vi "actuationIT6412w2110.vi"() -> ()   [LabVIEW 2023]
uses:
  IT64001/IT6400.lvlib
panel:
  out "error out 5":errorcluster
  in  "stop 5":bool
  out "Voltage 6":cluster{"Y":dbl[], "Y":dbl[]}[](graph)
  out "Voltage 6":dbl[](graph)
  out "Voltage 6":dbl[](array[numeric])
  out "error out 4":errorcluster
  out "Current time 4":timestamp
  in  "error in (no error) 3":errorcluster
  in  "VISA 2110 for voltage":refnum<visa-resource-name>
  out "Current through 330 ohm resistor'/mA 3":cluster{"Y":dbl[], "Y":dbl[]}[](graph)
  out "Voltage across 330 ohm resistor' 5":dbl[](graph)
  out "Voltage across 330 ohm resistor' 4":dbl[](array[numeric])
  in  "Filename 4":path caption="Filename"
  in  "Volt (0 V) 3":dbl min=-15.0 max=15.0 format="%.3g"
  in  "On/Off 3":bool
  in  "Pause/ms 3":i32=20
  out "Actual Voltage Level (V) 3":dbl[](array[numeric])
  out "Voltage'/V 3":dbl[](graph)
  in  "stop 3":bool
  out "Voltage'/V 2":cluster{"Y":dbl[], "Y":dbl[]}[](graph)
  in  "Filename 3":path caption="Filename"
  out "Current time 3":timestamp
  in  "period/s 2":i32
  in  "Boolean 2":bool
  in  "on time 2":dbl format="%#_13g"
  out "Voltage across 330 ohm resistor' 3":dbl[](array[numeric])
  out "Voltage across 330 ohm resistor' 2":dbl[](graph)
  out "Current through 330 ohm resistor'/mA 2":cluster{"Y":dbl[], "Y":dbl[]}[](graph)
  out "Current through 330 ohm resistor'/mA":cluster{"Y":dbl[], "Y":dbl[]}[](graph)
  out "Voltage across 330 ohm resistor'":dbl[](graph)
  out "Voltage across 330 ohm resistor'":dbl[](array[numeric])
  in  "Volt (0 V) 2":dbl min=-15.0 max=15.0 format="%.3g"
  in  "On/Off 2":bool
  in  "Pause/ms 2":i32=20
  out "Actual Voltage Level (V) 2":dbl[](array[numeric])
  out "Voltage'/V":dbl[](graph)
  in  "stop 2":bool
  out "Voltage'/V":cluster{"Y":dbl[], "Y":dbl[]}[](graph)
  in  "Filename 2":path caption="Filename"
  out "Current time 2":timestamp
  in  "period/s":i32
  in  "Boolean":bool
  in  "on time":dbl format="%#_13g"
  in  "Freq Sweep (1)\nCyclic voltammetry (2)\nSigGen (3)":i32 min=0 max=3 step=1
  in  "Camera":bool=TRUE
  out "Start time":timestamp
  out "current through 330ohm resistor/mA":cluster{"Y":dbl[], "Y":dbl[]}[](graph)
  out "Voltage across 330 ohm resistor":dbl[](graph)
  out "voltage across 330ohm resistor/V":dbl[](array[numeric])
  out "error out 3":errorcluster
  in  "error in (no error) 2":errorcluster
  in  "VISA 2110 for current":refnum<visa-resource-name>
  out "Timer":dbl
  in  "Countdown/s":i32=3
  out "Current time":timestamp
  in  "Filename":path
  out "Voltage/V":cluster{"Y":dbl[], "Y":dbl[]}[](graph)
  in  "stop":bool
  in  "Pause/ms":i32=100
  out "Voltage/V":dbl[](graph)
  out "Actual Voltage Level (V)":dbl[](array[numeric])
  in  "Sign":bool=TRUE
  in  "On/Off":bool
  in  "Volt (0 V)":dbl min=-15.0 max=15.0 format="%.3g"
  in  "Volt Limit (0 V)":dbl=9.0 min=0.0 max=15.0 format="%.3g"
  in  "Enable Volt Lim (T: Enable)":bool=TRUE
  in  "Curr Limit (0 A)":dbl=1.0 min=0.0 format="%.3g"
  in  "Enable Curr Lim (T: Enable)":bool=TRUE
  in  "Channel":i32=1 min=1 max=2
  in  "VOLT Range (0.0 v)":dbl=9.0 min=0.0 max=15.0 format="%.2g"
  in  "Enable OVP (T: Enable)":bool=TRUE
  in  "Reset":bool
  in  "Serial Configuration":T1={"Baud Rate"=9600, "Parity"=0, "Data Bits"=8, "Stop Bits"=10} {"Stop Bits" items=["1.0"=10, "1.5"=15, "2.0"=20]; "Data Bits" items=["7"=7, "8"=8]; "Parity" items=["None", "Odd", "Even", "Mark", "Space"]; "Baud Rate" items=["300"=300, "600"=600, "1200"=1200, "2400"=2400, "4800"=4800, "9600"=9600, "19200"=19200]}
  in  "Local/\nRemote":bool caption="Local/Remote"
  out "VISA resource name out":refnum<visa-resource-name>
  out "error out":errorcluster
  in  "error in (no error)":errorcluster
  in  "VISA resource name":refnum<visa-resource-name>
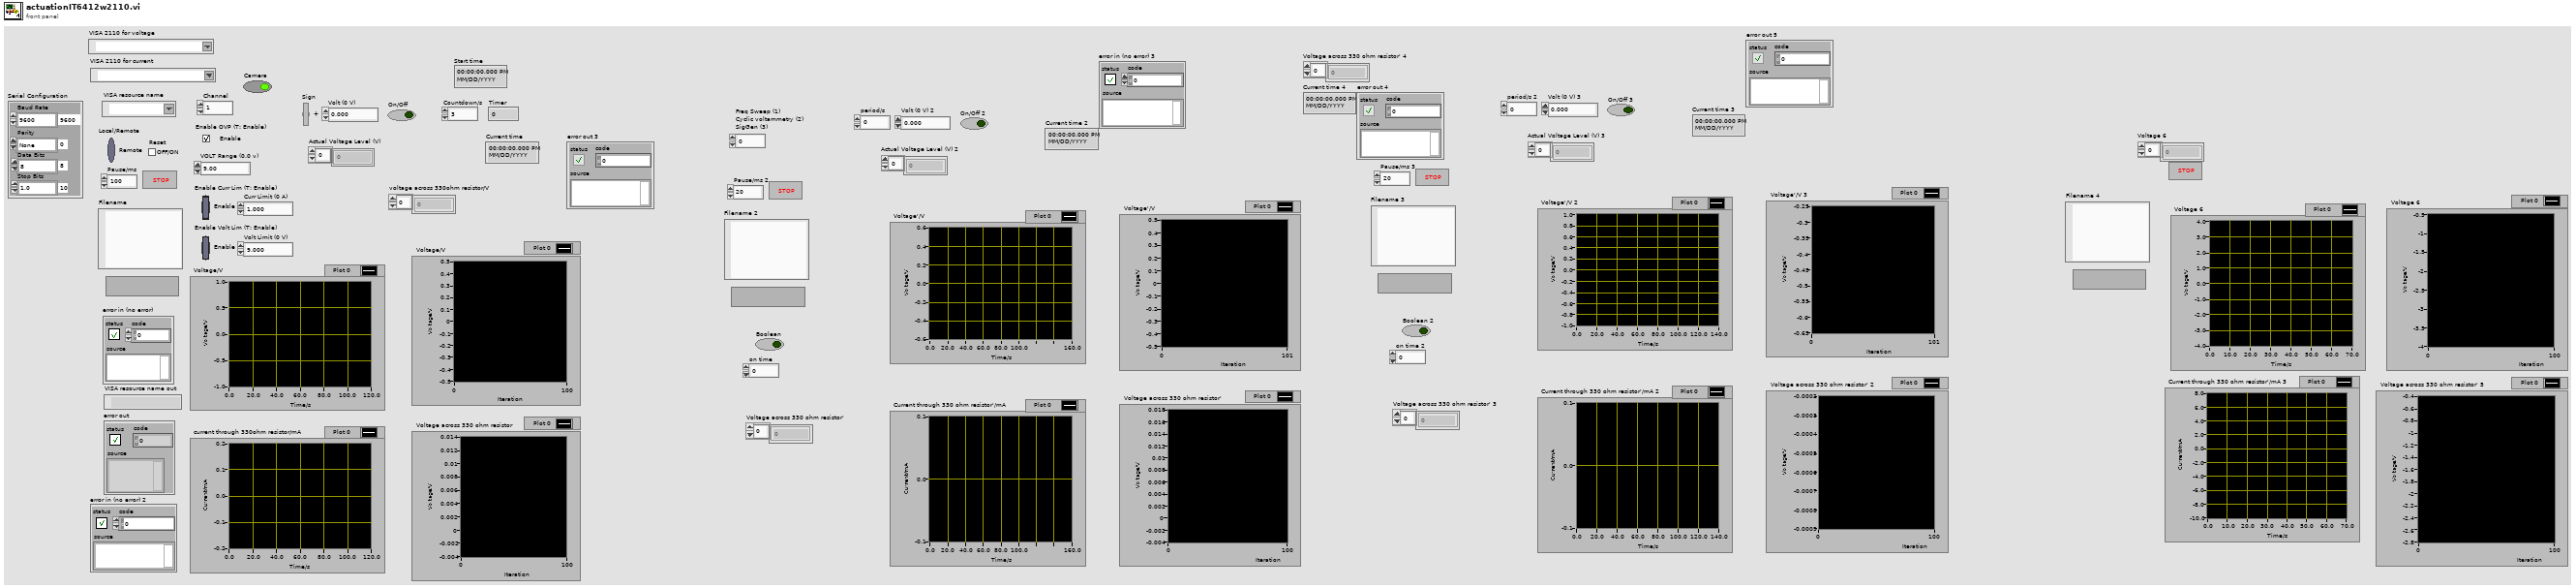
[diagram p1: front panel]
types:
  T1 = cluster{"Baud Rate":u32, "Parity":u16, "Data Bits":u16, "Stop Bits":u16}
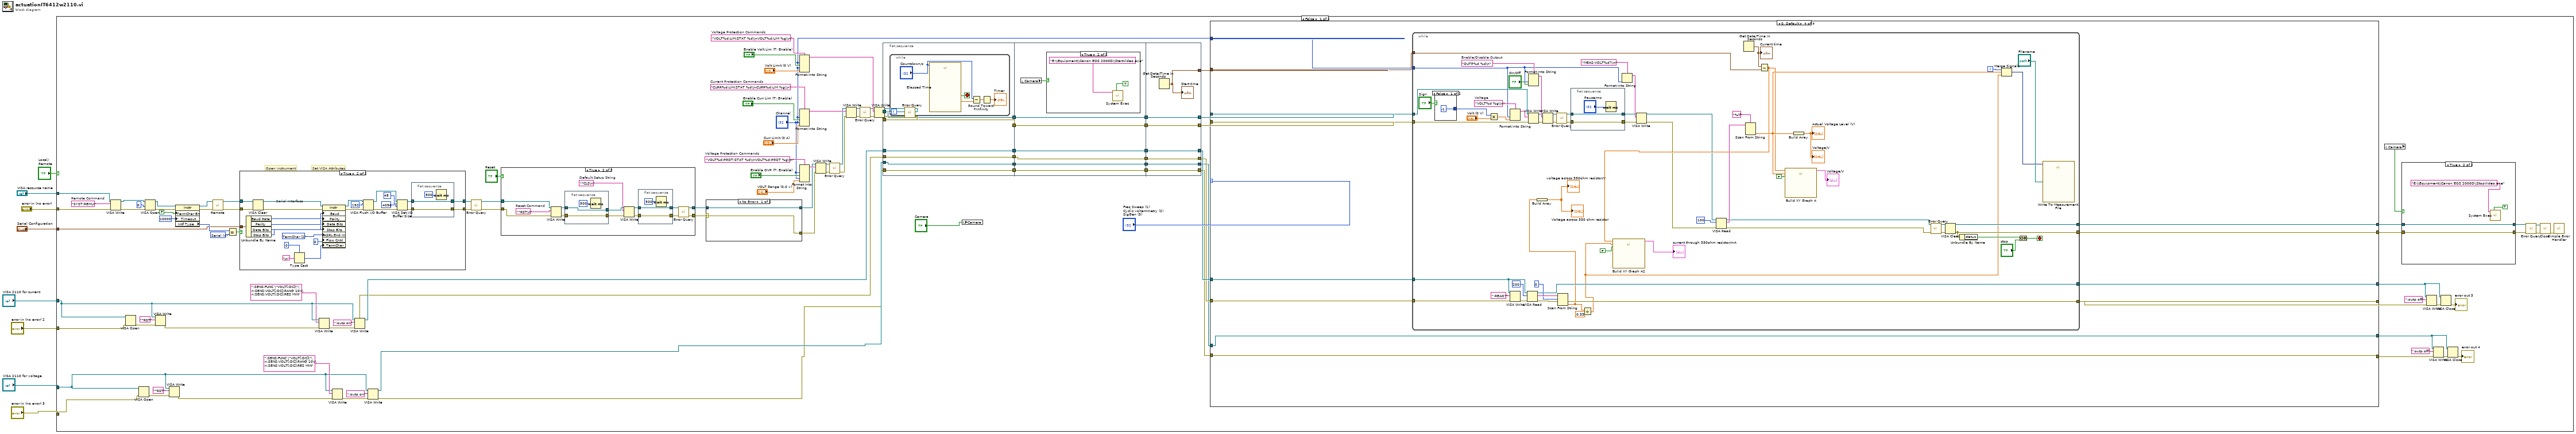
[diagram p0: block diagram]
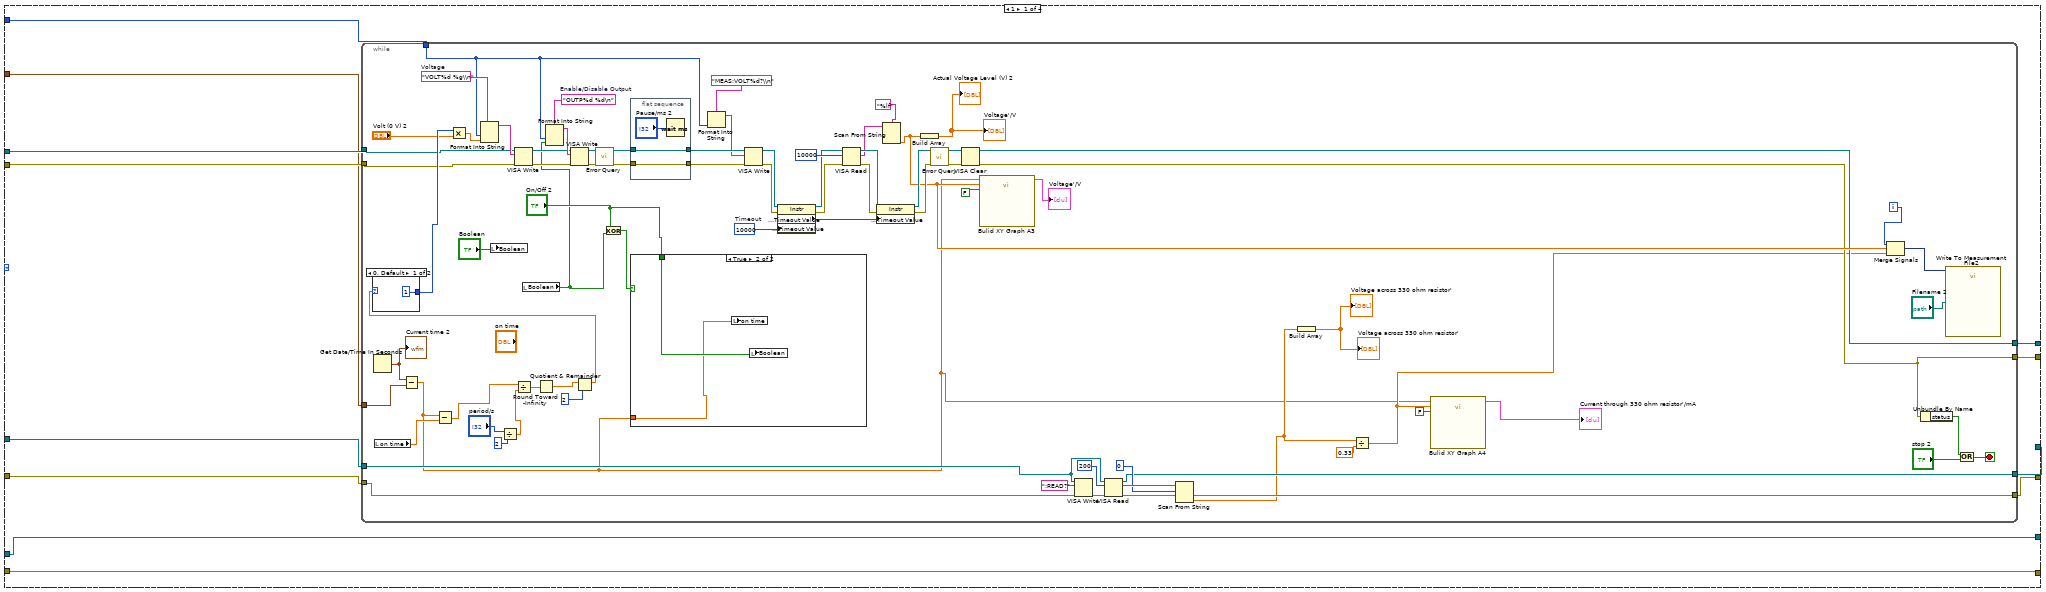
[diagram p2: hidden frame]
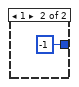
[diagram p4: hidden frame]
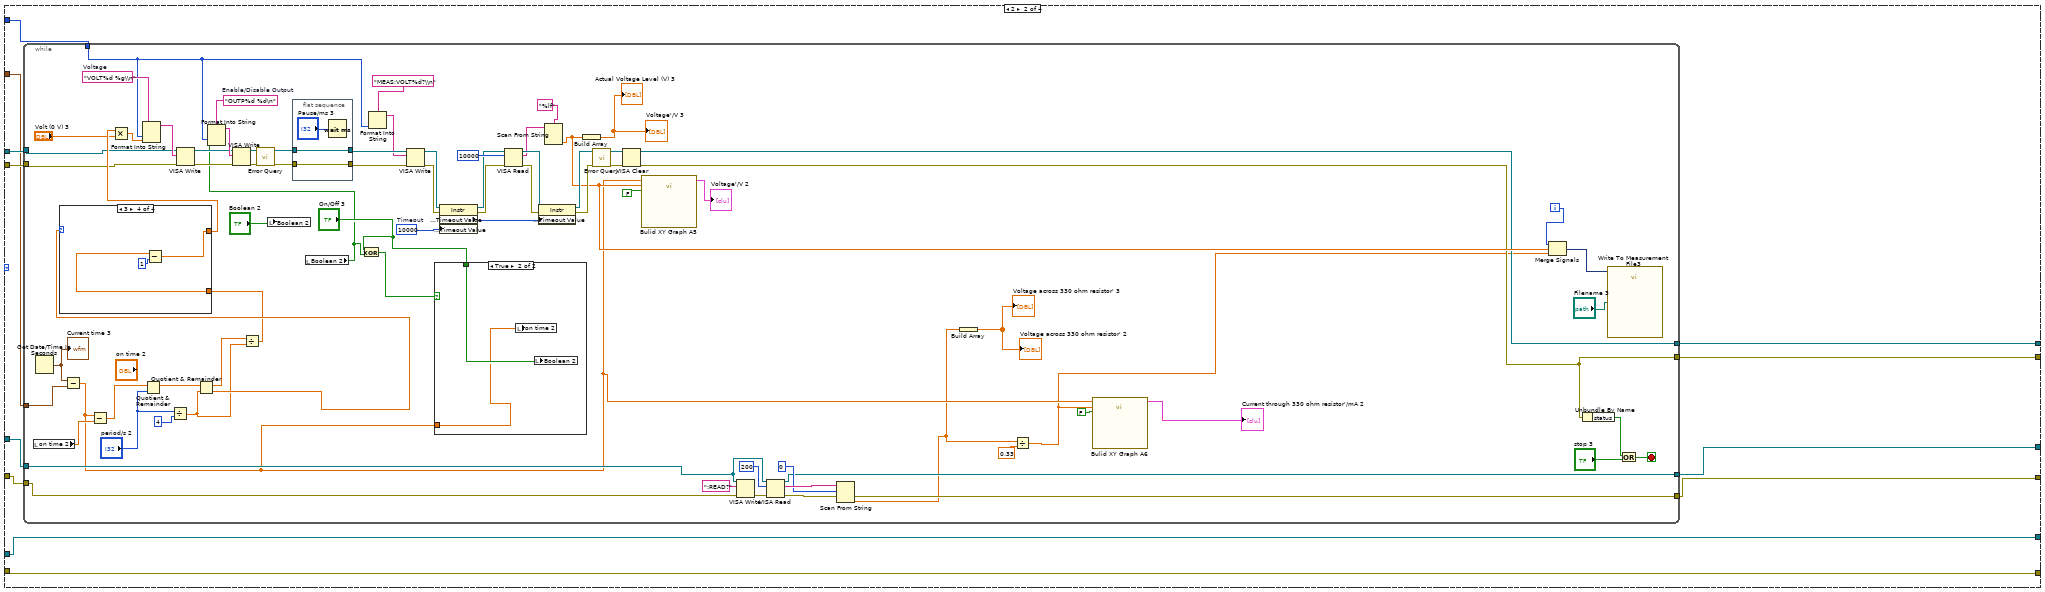
[diagram p5: hidden frame]
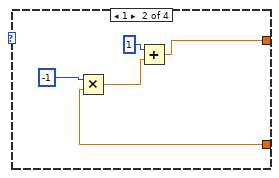
[diagram p8: hidden frame]
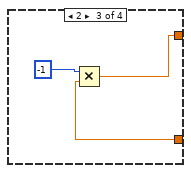
[diagram p9: hidden frame]
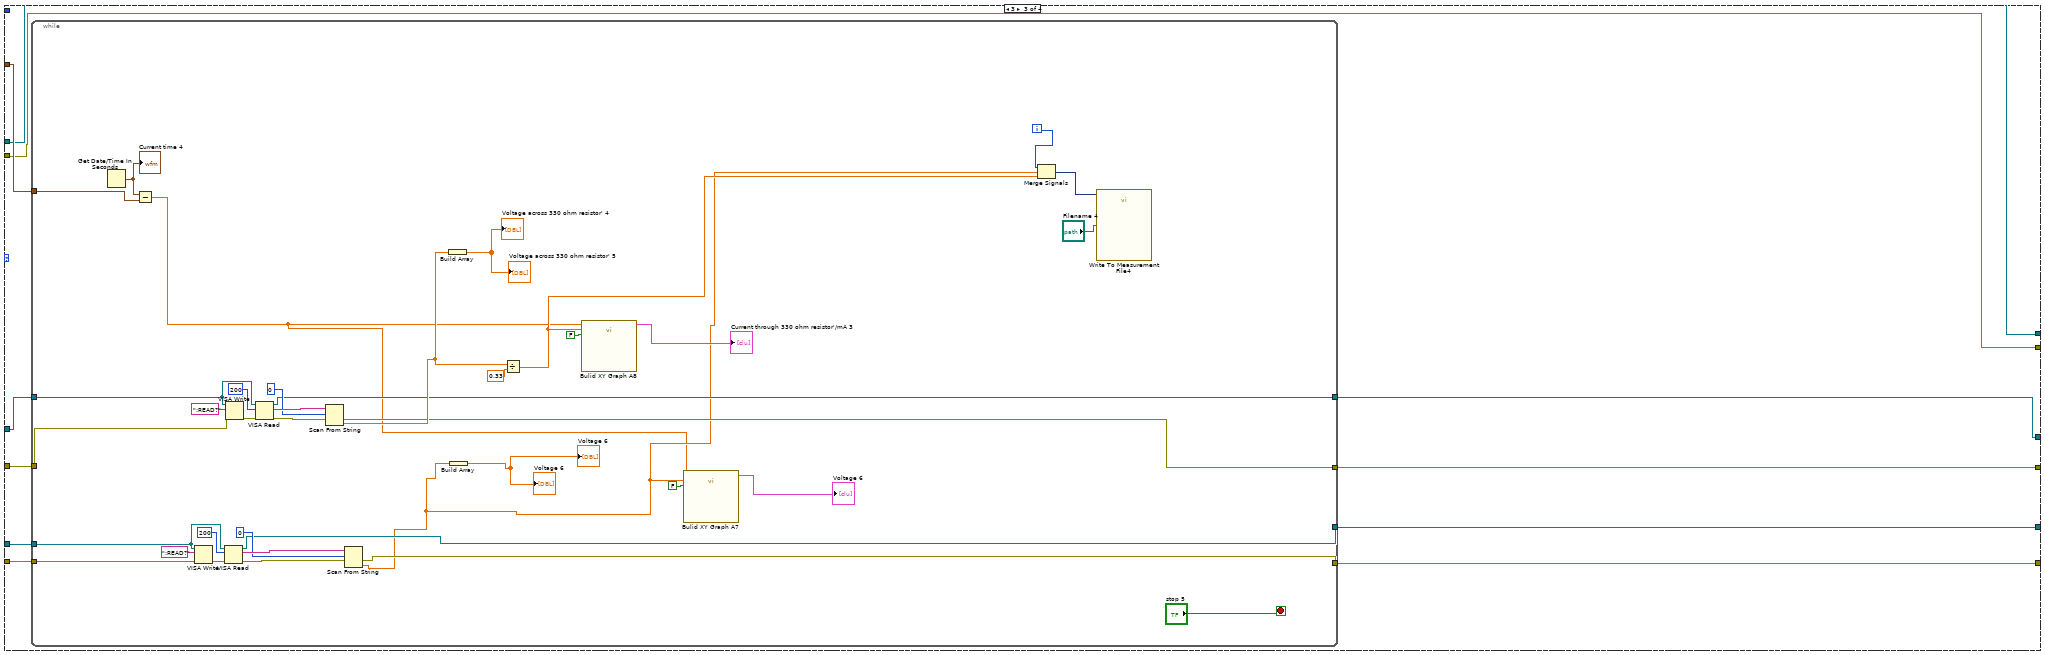
[diagram p10: hidden frame]
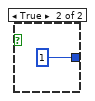
[diagram p11: hidden frame]
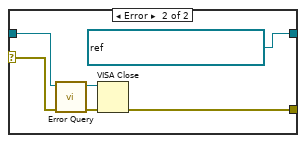
[diagram p14: hidden frame]
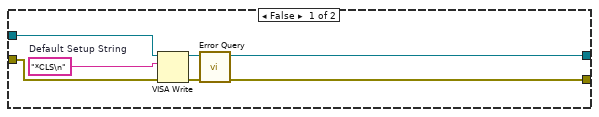
[diagram p15: hidden frame]
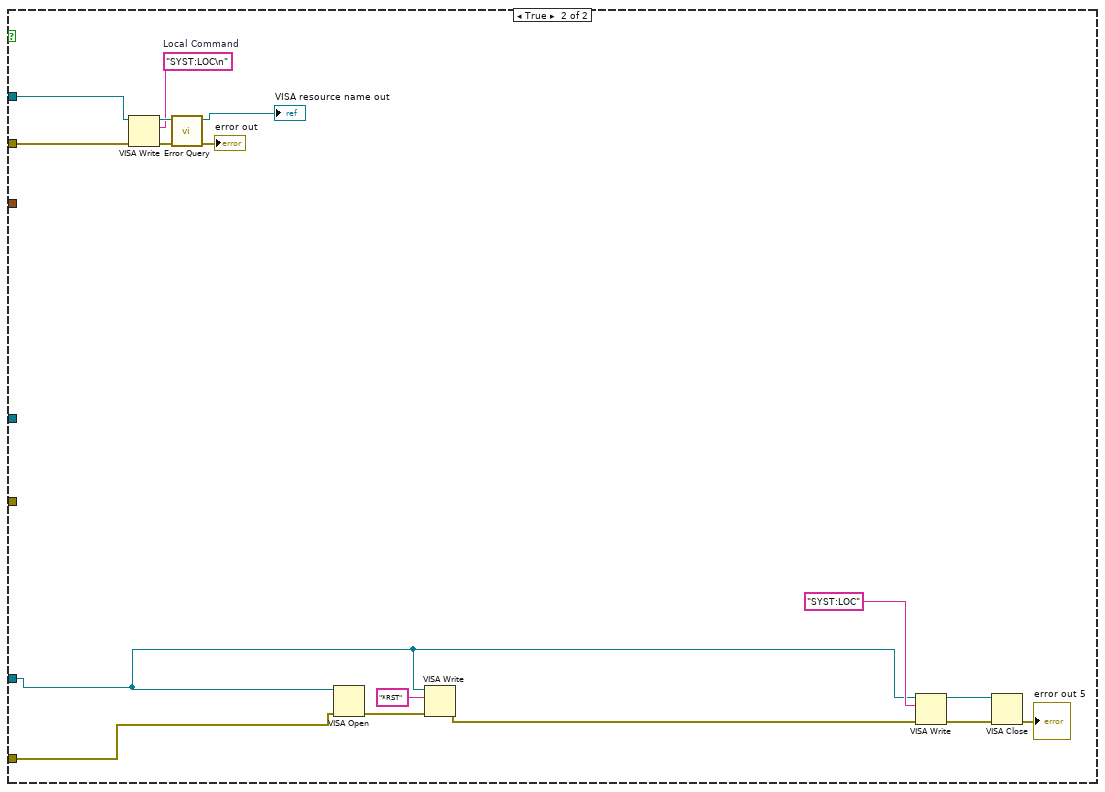
[diagram p17: hidden frame]
diagram:
  n1 = case shown="False" "Local/\nRemote" {
    tunnel: "VISA resource name" -> [w118 w562]
    tunnel: "error in (no error)" -> [w117 w561]
    tunnel: "Serial Configuration" -> [w102 _]
    tunnel: "VISA 2110 for current" -> [w56 _]
    tunnel: "error in (no error) 2" -> [w55 _]
    tunnel: "error in (no error) 3" -> [w31 w554]
    tunnel: "VISA 2110 for voltage" -> [w30 w555]
    frame False {
      w80 = "VOLT%d:LIM:STAT %d\\nVOLT%d:LIM %g\\n"  # Voltage Protection Commands
      w88 = "CURR%d:LIM:STAT %d\\nCURR%d:LIM %g\\n"  # Current Protection Commands
      w94 = "VOLT%d:PROT:STAT %d\\nVOLT%d:PROT %g\\n"  # Voltage Protection Commands
      w115 = u16 4 items=["GPIB"=1, "VXI"=2, "GPIB-VXI"=3, "Serial"=4, "PXI"=5, "TCPIP"=6, "USB"=7] ("Interface Information:Interface Type")
      w119 = "SYST:REM\n"  # Remote Command
      # "Set VISA Attributes"
      # "Open instrument"
      n2 = VISA Write(VISA resource name=w118, write buffer=w119, error in (no error)=w117) -> (VISA resource name out=w101:refnum<visa-resource-name>, error out=w100:errorcluster)  [unwired: 1 out]
      n3 = VISA Open(error in (no error)=w55, VISA resource name=w56) -> (error out=w59:errorcluster)  [unwired: 3 in, 1 out]
      n4 = VISA Open(error in (no error)=w31, VISA resource name=w30) -> (error out=w37:errorcluster)  [unwired: 3 in, 1 out]
      n5 = VISA Open(access mode=u32 0, error in (no error)=w100, VISA resource name=w101) -> (VISA resource name=w113:refnum<visa-resource-name>, error out=w112:errorcluster)  [unwired: 2 in]
      n6 = VISA Write(VISA resource name=w56, write buffer="*RST" ("数据"), error in (no error)=w59) -> (error out=w58:errorcluster)  [unwired: 2 out]
      n7 = VISA Write(VISA resource name=w30, write buffer="*RST" ("数据"), error in (no error)=w37) -> (error out=w36:errorcluster)  [unwired: 2 out]
      n8 = property class="Instr"(reference=w113, error in=w112, "TermChar En"=FALSE, "Timeout"=u32 10000 ("General Settings:Timeout Value")) -> (reference out=w107:refnum<visa-resource-name>, error out=w106:errorcluster, "Intf Type"=w103:u16)
      n9 = call "Remote.vi"("error in (no error)"=w106, "VISA resource name"=w107) -> ("error out"=w108:errorcluster, "VISA resource name out"=w109:refnum<visa-resource-name>)  [unwired: 8 in]
      n10 = Equal?(x=w103, y=w115) -> (x = y?=w116:bool)
      n11 = case shown="True" w116 {
        tunnel: [w521 w525] -> w111
        tunnel: [w522 w524] -> w110
        tunnel: w109 -> [w521 w540]
        tunnel: w108 -> [w522 w539]
        tunnel: w102 -> [_ w523]
        frame False {
          # "EDIT: Remove interfaces not supported by your instrument."
          # "GPIB, TCP/IP, and USB Interface"
        }
        frame True {
          w534 = u16 2 items=["None", "LastBit", "TermChar"] ("Serial Settings:Serial End Mode for Reads")
          # "Serial Interface"
          n12 = Unbundle By Name(w523) -> ("Baud Rate"=w536:u32, "Parity"=w533:u16, "Data Bits"=w532:u16, "Stop Bits"=w535:u16)
          n13 = VISA Clear(VISA resource name=w540, error in (no error)=w539) -> (VISA resource name out=w538:refnum<visa-resource-name>, error out=w537:errorcluster)
          n14 = Type Cast(type=u8 0, x="\n" ("Line Feed Constant")) -> (*(type *) &x=w530:u8)
          n15 = property class="Instr"(reference=w538, error in=w537, "Baud"=w536, "Parity"=w533, "Data Bits"=w532, "Stop Bits"=w535, "ASRL End In"=w534, "Flow Cntrl"=0, "TermChar"=w530) -> (reference out=w546:refnum<visa-resource-name>, error out=w547:errorcluster)
          n16 = VISA Flush I/O Buffer(VISA resource name=w546, mask (16)=u16 192, error in (no error)=w547) -> (VISA resource name out=w529:refnum<visa-resource-name>, error out=w528:errorcluster)
          n17 = VISA Set I/O Buffer Size(VISA resource name=w529, mask (16)=u16 48, size (4096)=u32 4096 ("size (0)"), error in (no error)=w528) -> (VISA resource name out=w527:refnum<visa-resource-name>, error out=w526:errorcluster)
          n18 = flat-sequence {
            tunnel: w527 -> [w550]
            tunnel: w526 -> [w549]
            tunnel: [w550] -> w525
            tunnel: [w549] -> w524
            frame #0 {
              n19 = Wait (ms)(milliseconds to wait=500) -> ()  [unwired: 1 out]
            }
          }
        }
      }
      n20 = VISA Write(VISA resource name=w56, write buffer=":SENS:FUNC \"VOLT[:DC]\"\n:SENS:VOLT[:DC]:RANG 10V\n:SENS:VOLT[:DC]:RES MIN" ("address string"), error in (no error)=w58) -> (error out=w57:errorcluster)  [unwired: 2 out]
      n21 = VISA Write(VISA resource name=w30, write buffer=":SENS:FUNC \"VOLT[:DC]\"\n:SENS:VOLT[:DC]:RANG 10V\n:SENS:VOLT[:DC]:RES MIN" ("address string"), error in (no error)=w36) -> (error out=w35:errorcluster)  [unwired: 2 out]
      n22 = VISA Write(VISA resource name=w56, write buffer=":outp on" ("数据"), error in (no error)=w57) -> (VISA resource name out=w23:refnum<visa-resource-name>, error out=w18:errorcluster)  [unwired: 1 out]
      n23 = VISA Write(VISA resource name=w30, write buffer=":outp on" ("数据"), error in (no error)=w35) -> (VISA resource name out=w14:refnum<visa-resource-name>, error out=w12:errorcluster)  [unwired: 1 out]
      n24 = call "Error Query.vi"("error in (no error)"=w110, "VISA resource name"=w111) -> ("error out"=w97:errorcluster, "VISA resource name out"=w98:refnum<visa-resource-name>)  [unwired: 6 in, 2 out]
      n25 = case shown="True" "Reset" {
        tunnel: w98 -> [w499 w509]
        tunnel: w97 -> [w497 w508]
        tunnel: [w495 w502] -> w96
        tunnel: [w494 w501] -> w95
        frame False {
          w500 = "*CLS\n"  # Default Setup String
          n26 = VISA Write(VISA resource name=w499, write buffer=w500, error in (no error)=w497) -> (VISA resource name out=w498:refnum<visa-resource-name>, error out=w496:errorcluster)  [unwired: 1 out]
          n27 = call "Error Query.vi"("error in (no error)"=w496, "VISA resource name"=w498) -> ("error out"=w494:errorcluster, "VISA resource name out"=w495:refnum<visa-resource-name>)  [unwired: 6 in, 2 out]
        }
        frame True {
          w505 = "*CLS\n"  # Default Setup String
          w514 = "*RST\n"  # Reset Command
          n28 = VISA Write(VISA resource name=w509, write buffer=w514, error in (no error)=w508) -> (VISA resource name out=w513:refnum<visa-resource-name>, error out=w512:errorcluster)  [unwired: 1 out]
          n29 = flat-sequence {
            tunnel: w513 -> [w520]
            tunnel: [w520] -> w507
            tunnel: w512 -> [w518]
            tunnel: [w518] -> w506
            frame #0 {
              n30 = Wait (ms)(milliseconds to wait=500) -> ()  [unwired: 1 out]
            }
          }
          n31 = VISA Write(VISA resource name=w507, write buffer=w505, error in (no error)=w506) -> (VISA resource name out=w504:refnum<visa-resource-name>, error out=w503:errorcluster)  [unwired: 1 out]
          n32 = flat-sequence {
            tunnel: w504 -> [w517]
            tunnel: [w517] -> w511
            tunnel: [w515] -> w510
            tunnel: w503 -> [w515]
            frame #0 {
              n33 = Wait (ms)(milliseconds to wait=500) -> ()  [unwired: 1 out]
            }
          }
          n34 = call "Error Query.vi"("error in (no error)"=w510, "VISA resource name"=w511) -> ("error out"=w501:errorcluster, "VISA resource name out"=w502:refnum<visa-resource-name>)  [unwired: 6 in, 2 out]
        }
      }
      n35 = case shown="No Error" w95 {
        selector: w95 -> [w486 w489]
        tunnel: w96 -> [w487 w490]
        tunnel: [w487 refnum<visa-resource-name> "USB0::0x2EC7::0x6412::800624011767410027::INSTR" ("VISA resource name out")] -> w61
        tunnel: [w486 w488] -> w60
        frame No Error {
        }
        frame Error {
          n36 = call "Error Query.vi"("error in (no error)"=w489, "VISA resource name"=w490) -> ("error out"=w492:errorcluster, "VISA resource name out"=w491:refnum<visa-resource-name>)  [unwired: 6 in, 2 out]
          n37 = VISA Close(VISA resource name=w491, error in (no error)=w492) -> (error out=w488:errorcluster)
        }
      }
      n38 = Format Into String(format string=w80, "Channel", "Enable Volt Lim (T: Enable)", "Channel", "Volt Limit (0 V)") -> (resulting string=w77:string)  [unwired: 2 in, 1 out]
      n39 = Format Into String(format string=w88, "Channel", "Enable Curr Lim (T: Enable)", "Channel", "Curr Limit (0 A)") -> (resulting string=w85:string)  [unwired: 2 in, 1 out]
      n40 = Format Into String(format string=w94, "Channel", "Enable OVP (T: Enable)", "Channel", "VOLT Range (0.0 v)") -> (resulting string=w91:string)  [unwired: 2 in, 1 out]
      n41 = VISA Write(VISA resource name=w61, write buffer=w91, error in (no error)=w60) -> (VISA resource name out=w92:refnum<visa-resource-name>, error out=w93:errorcluster)  [unwired: 1 out]
      n42 = call "Error Query.vi"("error in (no error)"=w93, "VISA resource name"=w92) -> ("error out"=w81:errorcluster, "VISA resource name out"=w82:refnum<visa-resource-name>)  [unwired: 6 in, 2 out]
      n43 = VISA Write(VISA resource name=w82, write buffer=w85, error in (no error)=w81) -> (VISA resource name out=w86:refnum<visa-resource-name>, error out=w87:errorcluster)  [unwired: 1 out]
      n44 = call "Error Query.vi"("error in (no error)"=w87, "VISA resource name"=w86) -> ("error out"=w73:errorcluster, "VISA resource name out"=w74:refnum<visa-resource-name>)  [unwired: 6 in, 2 out]
      n45 = VISA Write(VISA resource name=w74, write buffer=w77, error in (no error)=w73) -> (VISA resource name out=w78:refnum<visa-resource-name>, error out=w79:errorcluster)  [unwired: 1 out]
      n46 = flat-sequence {
        tunnel: w66 -> [w463]
        tunnel: w68 -> [w464]
        tunnel: [w464] -> w63
        tunnel: [w463] -> w62
        tunnel: [w462] -> w24
        tunnel: w23 -> [w462]
        tunnel: [w461] -> w20
        tunnel: w18 -> [w461]
        tunnel: w14 -> [w460]
        tunnel: [w460] -> w15
        tunnel: w12 -> [w459]
        tunnel: [w459] -> w10
        tunnel: w63 -> [w476]
        tunnel: w62 -> [w475]
        tunnel: [w476] -> w46
        tunnel: [w475] -> w45
        tunnel: w24 -> [w473]
        tunnel: [w473] -> w22
        tunnel: w20 -> [w472]
        tunnel: [w472] -> w19
        tunnel: [w471] -> w16
        tunnel: w15 -> [w471]
        tunnel: [w470] -> w11
        tunnel: w10 -> [w470]
        tunnel: [w483] -> w64
        tunnel: [w484] -> w65
        tunnel: [w485] -> w67
        tunnel: w46 -> [w485]
        tunnel: w45 -> [w484]
        tunnel: [w482] -> w21
        tunnel: w22 -> [w482]
        tunnel: [w481] -> w17
        tunnel: w19 -> [w481]
        tunnel: [w480] -> w13
        tunnel: w16 -> [w480]
        tunnel: [w479] -> w9
        tunnel: w11 -> [w479]
        frame #0 {
          n47 = while {
            stop <- w467 stop-if-true
            n48 = call "Elapsed Time"("Time Target (s)"="Countdown/s") -> ("Elapsed Time (s)"=w469:dbl, "Time has Elapsed"=w467:bool)  [unwired: 11 in, 6 out]
            n49 = Subtract(x="Countdown/s", y=w469) -> (x-y=w466:dbl)
            n50 = Round Toward +Infinity(x=w466) -> (ceil(x): smallest int >= x=→"Timer":dbl)
          }
        }
        frame #1 {
          n51 = local read "Camera"() -> (w474:bool)
          n52 = case shown="True" w474 {
            frame False {
            }
            frame True {
              n53 = call <vilib>:"System Exec.vi"("wait until completion? (T)"=TRUE, "command line"="E:\\Equipment\\Canon EOS 2000D\\StartVideo.exe") -> ()  [unwired: 6 in, 4 out]
            }
          }
        }
        frame #2 {
          n54 = Get Date/Time In Seconds() -> (seconds since 1Jan1904=w483:timestamp)
          "Start time" <- w483
        }
      }
      n55 = call "Error Query.vi"("error in (no error)"=w79, "VISA resource name"=w78) -> ("error out"=w66:errorcluster, "VISA resource name out"=w68:refnum<visa-resource-name>)  [unwired: 6 in, 2 out]
      n56 = local write "Camera"("Camera") -> ()
      n57 = case shown="0, Default" "Freq Sweep (1)\nCyclic voltammetry (2)\nSigGen (3)" {
        tunnel: "Channel" -> [w131 w227 _ w385]
        tunnel: w67 -> [w130 w229 w329 w384]
        tunnel: w65 -> [w129 w228 w328 w383]
        tunnel: w64 -> [w128 w226 w332 w382]
        tunnel: w21 -> [w125 w225 w336 w381]
        tunnel: w17 -> [w124 w224 w335 w380]
        tunnel: [w123 w221 w331 w379] -> w48
        tunnel: [w122 w220 w330 w378] -> w47
        tunnel: [w127 w223 w329 w377] -> w43
        tunnel: [w126 w222 w328 w376] -> w41
        tunnel: w13 -> [w121 w219 w334 w375]
        tunnel: w9 -> [w120 w218 w333 w374]
        tunnel: [w121 w219 w327 w375] -> w26
        tunnel: [w120 w218 w326 w374] -> w25
        frame 1 {
          n58 = while {
            tunnel: w131 -> [w140]
            tunnel: w130 -> [w168]
            tunnel: w129 -> [w167]
            tunnel: [w138] -> w126
            tunnel: [w139] -> w127
            tunnel: w128 -> [w157]
            tunnel: w125 -> [w145]
            tunnel: w124 -> [w144]
            tunnel: [w143] -> w123
            tunnel: [w142] -> w122
            i -> [w141]
            stop <- w177 stop-if-true
            w196 = u32 10000  # Timeout
            w203 = "VOLT%d %g\\n"  # Voltage
            w210 = "OUTP%d %d\n"  # Enable/Disable Output
            n59 = Get Date/Time In Seconds() -> (seconds since 1Jan1904=w170:timestamp)
            "Current time 2" <- w170
            n60 = local read "on time"() -> (w134:dbl)
            n61 = Subtract(x=w170, y=w157) -> (x-y=w133:dbl)
            n62 = Subtract(x=w133, y=w134) -> (x-y=w156:dbl)
            n63 = local write "Boolean"("Boolean") -> ()
            n64 = Divide(x="period/s", y=2) -> (x/y=w166:dbl)
            n65 = Divide(x=w156, y=w166) -> (x/y=w163:dbl)
            n66 = local read "Boolean"() -> (w132:bool)
            n67 = Round Toward -Infinity(1:w163) -> (0:w162:dbl)
            n68 = Format Into String(format string=w210, w140, w132) -> (resulting string=w207:string)  [unwired: 2 in, 1 out]
            n69 = Quotient & Remainder(x=w162, y=2) -> (x-y*floor(x/y)=w160:dbl)  [unwired: 1 out]
            n70 = case shown="0, Default" w160 {
              tunnel: [1 -1] -> w200
              frame 0, Default {
              }
              frame 1 {
              }
            }
            n71 = Multiply(x=w200, y="Volt (0 V) 2") -> (x*y=w198:dbl)
            n72 = Format Into String(format string=w203, w140, w198) -> (resulting string=w204:string)  [unwired: 2 in, 1 out]
            n73 = VISA Write(VISA resource name=w168, write buffer=w204, error in (no error)=w167) -> (VISA resource name out=w205:refnum<visa-resource-name>, error out=w206:errorcluster)  [unwired: 1 out]
            n74 = VISA Write(VISA resource name=w205, write buffer=w207, error in (no error)=w206) -> (VISA resource name out=w209:refnum<visa-resource-name>, error out=w208:errorcluster)  [unwired: 1 out]
            n75 = call "Error Query.vi"("error in (no error)"=w208, "VISA resource name"=w209) -> ("error out"=w201:errorcluster, "VISA resource name out"=w202:refnum<visa-resource-name>)  [unwired: 6 in, 2 out]
            n76 = Exclusive Or(1:w132, 2:"On/Off 2") -> (0:w158:bool)
            n77 = flat-sequence {
              tunnel: [w216] -> w182
              tunnel: w202 -> [w216]
              tunnel: w201 -> [w215]
              tunnel: [w215] -> w181
              frame #0 {
                n78 = Wait (ms)(milliseconds to wait="Pause/ms 2") -> ()  [unwired: 1 out]
              }
            }
            n79 = case shown="True" w158 {
              tunnel: "On/Off 2" -> [_ w212]
              tunnel: w133 -> [_ w211]
              frame False {
              }
              frame True {
                n80 = local write "on time"(w211) -> ()
                n81 = local write "Boolean"(w212) -> ()
              }
            }
            n82 = Format Into String(format string="MEAS:VOLT%d?\\n", w140) -> (resulting string=w179:string)  [unwired: 2 in, 1 out]
            n83 = VISA Write(VISA resource name=w182, write buffer=w179, error in (no error)=w181) -> (VISA resource name out=w193:refnum<visa-resource-name>, error out=w192:errorcluster)  [unwired: 1 out]
            n84 = property class="Instr"(reference=w193, error in=w192, "General Settings:Timeout Value"=w196) -> (reference out=w191:refnum<visa-resource-name>, error out=w190:errorcluster, "General Settings:Timeout Value"=w187:u32)
            n85 = VISA Read(VISA resource name=w191, byte count=10000, error in (no error)=w190) -> (VISA resource name out=w188:refnum<visa-resource-name>, read buffer=w183:string, error out=w189:errorcluster)  [unwired: 1 out]
            n86 = property class="Instr"(reference=w188, error in=w189, "General Settings:Timeout Value"=w187) -> (reference out=w195:refnum<visa-resource-name>, error out=w194:errorcluster)
            n87 = Scan From String(format string="%lf", input string=w183) -> (output 1=w169:dbl)  [unwired: 3 in, 3 out]
            n88 = Build Array(w169) -> (→"Actual Voltage Level (V) 2" →"Voltage'/V":dbl[])
            n89 = call "Error Query.vi"("error in (no error)"=w194, "VISA resource name"=w195) -> ("error out"=w185:errorcluster, "VISA resource name out"=w186:refnum<visa-resource-name>)  [unwired: 6 in, 2 out]
            n90 = VISA Clear(VISA resource name=w186, error in (no error)=w185) -> (VISA resource name out=w139:refnum<visa-resource-name>, error out=w138:errorcluster)
            n91 = call "Bulid XY Graph A3"("Reset"=FALSE, "Y Input"=w169, "X Input"=w133) -> ("XY Graph"=→"Voltage'/V":cluster{"X":dbl[], "Y":dbl[]}[])  [unwired: 7 in, 1 out]
            n92 = VISA Write(VISA resource name=w145, write buffer=":READ?" ("数据"), error in (no error)=w144) -> (error out=w152:errorcluster)  [unwired: 2 out]
            n93 = VISA Read(VISA resource name=w145, byte count=200 ("字节总数"), error in (no error)=w152) -> (VISA resource name out=w143:refnum<visa-resource-name>, read buffer=w154:string, error out=w153:errorcluster)  [unwired: 1 out]
            n94 = Scan From String(input string=w154, initial scan location=u32 0 ("初始扫描位置"), error in=w153) -> (error out=w142:errorcluster, output 1=w137:dbl)  [unwired: 2 in, 2 out]
            n95 = Build Array(w137) -> (→"Voltage across 330 ohm resistor'" →"Voltage across 330 ohm resistor'":dbl[])
            n96 = Divide(x=w137, y=0.33) -> (x/y=w135:dbl)
            n97 = call "Bulid XY Graph A4"("Reset"=FALSE, "Y Input"=w135, "X Input"=w133) -> ("XY Graph"=→"Current through 330 ohm resistor'/mA":cluster{"X":dbl[], "Y":dbl[]}[])  [unwired: 7 in, 1 out]
            n98 = Merge Signals(w141, w169, w135) -> (w173:dynamicdata)
            n99 = Unbundle By Name(w138) -> ("status"=w178:bool)
            n100 = call "Write To Measurement File2"("Signals"=w173, "Filename"="Filename 2") -> ()  [unwired: 15 in, 3 out]
            n101 = Or(x=w178, y="stop 2") -> (x .or. y?=w177:bool)
          }
        }
        frame 2 {
          n102 = while {
            tunnel: w227 -> [w246]
            tunnel: w229 -> [w266]
            tunnel: w228 -> [w265]
            tunnel: [w244] -> w222
            tunnel: [w245] -> w223
            tunnel: w226 -> [w262]
            tunnel: w225 -> [w251]
            tunnel: w224 -> [w250]
            tunnel: [w249] -> w221
            tunnel: [w248] -> w220
            i -> [w247]
            stop <- w275 stop-if-true
            w294 = u32 10000  # Timeout
            w301 = "VOLT%d %g\\n"  # Voltage
            w308 = "OUTP%d %d\n"  # Enable/Disable Output
            n103 = local read "on time 2"() -> (w243:dbl)
            n104 = Get Date/Time In Seconds() -> (seconds since 1Jan1904=w268:timestamp)
            "Current time 3" <- w268
            n105 = Subtract(x=w268, y=w262) -> (x-y=w242:dbl)
            n106 = Subtract(x=w242, y=w243) -> (x-y=w240:dbl)
            n107 = Quotient & Remainder(x=w240, y="period/s 2") -> (x-y*floor(x/y)=w239:dbl)  [unwired: 1 out]
            n108 = Divide(x="period/s 2", y=4) -> (x/y=w234:dbl)
            n109 = Quotient & Remainder(x=w239, y=w234) -> (x-y*floor(x/y)=w236:dbl, floor(x/y)=w237:dbl)
            n110 = Divide(x=w236, y=w234) -> (x/y=w233:dbl)
            n111 = case shown="3" w237 {
              tunnel: [w311 w312 w319 w320] -> w298
              tunnel: w233 -> [w311 w315 w318 w322]
              frame 0, Default {
              }
              frame 1 {
                n112 = Multiply(x=-1, y=w315) -> (x*y=w314:dbl)
                n113 = Add(x=1, y=w314) -> (x+y=w312:dbl)
              }
              frame 2 {
                n114 = Multiply(x=-1, y=w318) -> (x*y=w319:dbl)
              }
              frame 3 {
                n115 = Subtract(x=w322, y=1) -> (x-y=w320:dbl)
              }
            }
            n116 = Multiply(x=w298, y="Volt (0 V) 3") -> (x*y=w296:dbl)
            n117 = Format Into String(format string=w301, w246, w296) -> (resulting string=w302:string)  [unwired: 2 in, 1 out]
            n118 = VISA Write(VISA resource name=w266, write buffer=w302, error in (no error)=w265) -> (VISA resource name out=w303:refnum<visa-resource-name>, error out=w304:errorcluster)  [unwired: 1 out]
            n119 = local write "Boolean 2"("Boolean 2") -> ()
            n120 = flat-sequence {
              tunnel: [w324] -> w280
              tunnel: w300 -> [w324]
              tunnel: w299 -> [w323]
              tunnel: [w323] -> w279
              frame #0 {
                n121 = Wait (ms)(milliseconds to wait="Pause/ms 3") -> ()  [unwired: 1 out]
              }
            }
            n122 = local read "Boolean 2"() -> (w241:bool)
            n123 = Format Into String(format string=w308, w246, w241) -> (resulting string=w305:string)  [unwired: 2 in, 1 out]
            n124 = VISA Write(VISA resource name=w303, write buffer=w305, error in (no error)=w304) -> (VISA resource name out=w307:refnum<visa-resource-name>, error out=w306:errorcluster)  [unwired: 1 out]
            n125 = call "Error Query.vi"("error in (no error)"=w306, "VISA resource name"=w307) -> ("error out"=w299:errorcluster, "VISA resource name out"=w300:refnum<visa-resource-name>)  [unwired: 6 in, 2 out]
            n126 = Exclusive Or(1:w241, 2:"On/Off 3") -> (0:w263:bool)
            n127 = Format Into String(format string="MEAS:VOLT%d?\\n", w246) -> (resulting string=w277:string)  [unwired: 2 in, 1 out]
            n128 = VISA Write(VISA resource name=w280, write buffer=w277, error in (no error)=w279) -> (VISA resource name out=w291:refnum<visa-resource-name>, error out=w290:errorcluster)  [unwired: 1 out]
            n129 = case shown="True" w263 {
              tunnel: "On/Off 3" -> [_ w310]
              tunnel: w242 -> [_ w309]
              frame False {
              }
              frame True {
                n130 = local write "on time 2"(w309) -> ()
                n131 = local write "Boolean 2"(w310) -> ()
              }
            }
            n132 = property class="Instr"(reference=w291, error in=w290, "General Settings:Timeout Value"=w294) -> (reference out=w289:refnum<visa-resource-name>, error out=w288:errorcluster, "General Settings:Timeout Value"=w285:u32)
            n133 = VISA Read(VISA resource name=w289, byte count=10000, error in (no error)=w288) -> (VISA resource name out=w286:refnum<visa-resource-name>, read buffer=w281:string, error out=w287:errorcluster)  [unwired: 1 out]
            n134 = property class="Instr"(reference=w286, error in=w287, "General Settings:Timeout Value"=w285) -> (reference out=w293:refnum<visa-resource-name>, error out=w292:errorcluster)
            n135 = Scan From String(format string="%lf", input string=w281) -> (output 1=w267:dbl)  [unwired: 3 in, 3 out]
            n136 = Build Array(w267) -> (→"Actual Voltage Level (V) 3" →"Voltage'/V 3":dbl[])
            n137 = call "Error Query.vi"("error in (no error)"=w292, "VISA resource name"=w293) -> ("error out"=w283:errorcluster, "VISA resource name out"=w284:refnum<visa-resource-name>)  [unwired: 6 in, 2 out]
            n138 = VISA Clear(VISA resource name=w284, error in (no error)=w283) -> (VISA resource name out=w245:refnum<visa-resource-name>, error out=w244:errorcluster)
            n139 = call "Bulid XY Graph A5"("Reset"=FALSE, "Y Input"=w267, "X Input"=w242) -> ("XY Graph"=→"Voltage'/V 2":cluster{"X":dbl[], "Y":dbl[]}[])  [unwired: 7 in, 1 out]
            n140 = VISA Write(VISA resource name=w251, write buffer=":READ?" ("数据"), error in (no error)=w250) -> (error out=w258:errorcluster)  [unwired: 2 out]
            n141 = VISA Read(VISA resource name=w251, byte count=200 ("字节总数"), error in (no error)=w258) -> (VISA resource name out=w249:refnum<visa-resource-name>, read buffer=w260:string, error out=w259:errorcluster)  [unwired: 1 out]
            n142 = Scan From String(input string=w260, initial scan location=u32 0 ("初始扫描位置"), error in=w259) -> (error out=w248:errorcluster, output 1=w230:dbl)  [unwired: 2 in, 2 out]
            n143 = Build Array(w230) -> (→"Voltage across 330 ohm resistor' 3" →"Voltage across 330 ohm resistor' 2":dbl[])
            n144 = Divide(x=w230, y=0.33) -> (x/y=w231:dbl)
            n145 = call "Bulid XY Graph A6"("Reset"=FALSE, "Y Input"=w231, "X Input"=w242) -> ("XY Graph"=→"Current through 330 ohm resistor'/mA 2":cluster{"X":dbl[], "Y":dbl[]}[])  [unwired: 7 in, 1 out]
            n146 = Merge Signals(w247, w267, w231) -> (w271:dynamicdata)
            n147 = Unbundle By Name(w244) -> ("status"=w276:bool)
            n148 = call "Write To Measurement File3"("Signals"=w271, "Filename"="Filename 3") -> ()  [unwired: 15 in, 3 out]
            n149 = Or(x=w276, y="stop 3") -> (x .or. y?=w275:bool)
          }
        }
        frame 3 {
          n150 = while {
            tunnel: w336 -> [w359]
            tunnel: w335 -> [w358]
            tunnel: w334 -> [w351]
            tunnel: w333 -> [w350]
            tunnel: w332 -> [w348]
            tunnel: [w347] -> w331
            tunnel: [w346] -> w330
            tunnel: [w345] -> w327
            tunnel: [w344] -> w326
            i -> [w339]
            stop <- "stop 5" stop-if-true
            n151 = Get Date/Time In Seconds() -> (seconds since 1Jan1904=w349:timestamp)
            "Current time 4" <- w349
            n152 = Subtract(x=w349, y=w348) -> (x-y=w337:dbl)
            n153 = VISA Write(VISA resource name=w351, write buffer=":READ?" ("数据"), error in (no error)=w350) -> (error out=w355:errorcluster)  [unwired: 2 out]
            n154 = VISA Read(VISA resource name=w351, byte count=200 ("字节总数"), error in (no error)=w355) -> (VISA resource name out=w345:refnum<visa-resource-name>, read buffer=w357:string, error out=w356:errorcluster)  [unwired: 1 out]
            n155 = VISA Write(VISA resource name=w359, write buffer=":READ?" ("数据"), error in (no error)=w358) -> (error out=w369:errorcluster)  [unwired: 2 out]
            n156 = VISA Read(VISA resource name=w359, byte count=200 ("字节总数"), error in (no error)=w369) -> (VISA resource name out=w347:refnum<visa-resource-name>, read buffer=w371:string, error out=w370:errorcluster)  [unwired: 1 out]
            n157 = Scan From String(input string=w371, initial scan location=u32 0 ("初始扫描位置"), error in=w370) -> (error out=w346:errorcluster, output 1=w362:dbl)  [unwired: 2 in, 2 out]
            n158 = Scan From String(input string=w357, initial scan location=u32 0 ("初始扫描位置"), error in=w356) -> (error out=w344:errorcluster, output 1=w340:dbl)  [unwired: 2 in, 2 out]
            n159 = Build Array(w362) -> (→"Voltage across 330 ohm resistor' 4" →"Voltage across 330 ohm resistor' 5":dbl[])
            n160 = Build Array(w340) -> (→"Voltage 6" →"Voltage 6":dbl[])
            n161 = Divide(x=w362, y=0.33) -> (x/y=w360:dbl)
            n162 = call "Bulid XY Graph A8"("Reset"=FALSE, "Y Input"=w360, "X Input"=w337) -> ("XY Graph"=→"Current through 330 ohm resistor'/mA 3":cluster{"X":dbl[], "Y":dbl[]}[])  [unwired: 7 in, 1 out]
            n163 = call "Bulid XY Graph A7"("Reset"=FALSE, "Y Input"=w340, "X Input"=w337) -> ("XY Graph"=→"Voltage 6":cluster{"X":dbl[], "Y":dbl[]}[])  [unwired: 7 in, 1 out]
            n164 = Merge Signals(w339, w340, w360) -> (w373:dynamicdata)
            n165 = call "Write To Measurement File4"("Signals"=w373, "Filename"="Filename 4") -> ()  [unwired: 15 in, 3 out]
          }
        }
        frame 0, Default {
          n166 = while {
            tunnel: w385 -> [w423]
            tunnel: w384 -> [w411]
            tunnel: w383 -> [w410]
            tunnel: [w409] -> w376
            tunnel: [w408] -> w377
            tunnel: w382 -> [w414]
            tunnel: w381 -> [w401]
            tunnel: w380 -> [w400]
            tunnel: [w399] -> w379
            tunnel: [w398] -> w378
            i -> [w412]
            stop <- w421 stop-if-true
            w440 = "VOLT%d %g\\n"  # Voltage
            w447 = "OUTP%d %d\n"  # Enable/Disable Output
            n167 = case shown="False" "Sign" {
              tunnel: [-1 1] -> w435
              frame False {
              }
              frame True {
              }
            }
            n168 = Multiply(x=w435, y="Volt (0 V)") -> (x*y=w433:dbl)
            n169 = Format Into String(format string=w440, w423, w433) -> (resulting string=w441:string)  [unwired: 2 in, 1 out]
            n170 = VISA Write(VISA resource name=w401, write buffer=":READ?" ("数据"), error in (no error)=w400) -> (error out=w405:errorcluster)  [unwired: 2 out]
            n171 = VISA Read(VISA resource name=w401, byte count=200 ("字节总数"), error in (no error)=w405) -> (VISA resource name out=w399:refnum<visa-resource-name>, read buffer=w407:string, error out=w406:errorcluster)  [unwired: 1 out]
            n172 = Format Into String(format string=w447, w423, "On/Off") -> (resulting string=w444:string)  [unwired: 2 in, 1 out]
            n173 = VISA Write(VISA resource name=w411, write buffer=w441, error in (no error)=w410) -> (VISA resource name out=w442:refnum<visa-resource-name>, error out=w443:errorcluster)  [unwired: 1 out]
            n174 = VISA Write(VISA resource name=w442, write buffer=w444, error in (no error)=w443) -> (VISA resource name out=w446:refnum<visa-resource-name>, error out=w445:errorcluster)  [unwired: 1 out]
            n175 = call "Error Query.vi"("error in (no error)"=w445, "VISA resource name"=w446) -> ("error out"=w437:errorcluster, "VISA resource name out"=w438:refnum<visa-resource-name>)  [unwired: 6 in, 2 out]
            n176 = Scan From String(input string=w407, initial scan location=u32 0 ("初始扫描位置"), error in=w406) -> (error out=w398:errorcluster, output 1=w386:dbl)  [unwired: 2 in, 2 out]
            n177 = Build Array(w386) -> (→"voltage across 330ohm resistor/V" →"Voltage across 330 ohm resistor":dbl[])
            n178 = flat-sequence {
              tunnel: [w451] -> w429
              tunnel: w438 -> [w451]
              tunnel: w437 -> [w450]
              tunnel: [w450] -> w428
              frame #0 {
                n179 = Wait (ms)(milliseconds to wait="Pause/ms") -> ()  [unwired: 1 out]
              }
            }
            n180 = Divide(x=w386, y=0.33) -> (x/y=w387:dbl)
            n181 = Format Into String(format string="MEAS:VOLT%d?\\n", w423) -> (resulting string=w426:string)  [unwired: 2 in, 1 out]
            n182 = VISA Write(VISA resource name=w429, write buffer=w426, error in (no error)=w428) -> (VISA resource name out=w392:refnum<visa-resource-name>, error out=w391:errorcluster)  [unwired: 1 out]
            n183 = VISA Read(VISA resource name=w392, byte count=100, error in (no error)=w391) -> (VISA resource name out=w390:refnum<visa-resource-name>, read buffer=w430:string, error out=w389:errorcluster)  [unwired: 1 out]
            n184 = Get Date/Time In Seconds() -> (seconds since 1Jan1904=w415:timestamp)
            "Current time" <- w415
            n185 = Scan From String(format string="%lf", input string=w430) -> (output 1=w413:dbl)  [unwired: 3 in, 3 out]
            n186 = Subtract(x=w415, y=w414) -> (x-y=w393:dbl)
            n187 = call "Bulid XY Graph A2"("Reset"=FALSE, "Y Input"=w387, "X Input"=w393) -> ("XY Graph"=→"current through 330ohm resistor/mA":cluster{"X":dbl[], "Y":dbl[]}[])  [unwired: 7 in, 1 out]
            n188 = call "Bulid XY Graph A"("Reset"=FALSE, "Y Input"=w413, "X Input"=w393) -> ("XY Graph"=→"Voltage/V":cluster{"X":dbl[], "Y":dbl[]}[])  [unwired: 7 in, 1 out]
            n189 = Build Array(w413) -> (→"Actual Voltage Level (V)" →"Voltage/V":dbl[])
            n190 = call "Error Query.vi"("error in (no error)"=w389, "VISA resource name"=w390) -> ("error out"=w424:errorcluster, "VISA resource name out"=w425:refnum<visa-resource-name>)  [unwired: 6 in, 2 out]
            n191 = VISA Clear(VISA resource name=w425, error in (no error)=w424) -> (VISA resource name out=w408:refnum<visa-resource-name>, error out=w409:errorcluster)
            n192 = Unbundle By Name(w409) -> ("status"=w422:bool)
            n193 = Merge Signals(w412, w413, w387) -> (w417:dynamicdata)
            n194 = Or(x=w422, y="stop") -> (x .or. y?=w421:bool)
            n195 = call "Write To Measurement File"("Signals"=w417, "Filename"="Filename") -> ()  [unwired: 15 in, 3 out]
          }
        }
      }
      n196 = local read "Camera"() -> (w39:bool)
      n197 = case shown="True" w39 {
        tunnel: [w454 w456] -> w42
        tunnel: w43 -> [w454 w456]
        tunnel: w41 -> [w453 w455]
        tunnel: [w453 w455] -> w40
        frame False {
        }
        frame True {
          n198 = call <vilib>:"System Exec.vi"("wait until completion? (T)"=TRUE, "command line"="E:\\Equipment\\Canon EOS 2000D\\StopVideo.exe") -> ()  [unwired: 6 in, 4 out]
        }
      }
      n199 = VISA Write(VISA resource name=w48, write buffer=":outp off" ("数据"), error in (no error)=w47) -> (error out=w50:errorcluster)  [unwired: 2 out]
      n200 = VISA Write(VISA resource name=w26, write buffer=":outp off" ("数据"), error in (no error)=w25) -> (error out=w28:errorcluster)  [unwired: 2 out]
      n201 = VISA Close(VISA resource name=w48, error in (no error)=w50) -> (error out=→"error out 3":errorcluster)
      n202 = VISA Close(VISA resource name=w26, error in (no error)=w28) -> (error out=→"error out 4":errorcluster)
      n203 = call "Error Query.vi"("error in (no error)"=w40, "VISA resource name"=w42) -> ("error out"=w71:errorcluster, "VISA resource name out"=w70:refnum<visa-resource-name>)  [unwired: 6 in, 2 out]
      n204 = call "Close.vi"("error in (no error)"=w71, "VISA resource name"=w70) -> ("error out"=w69:errorcluster)  [unwired: 9 in]
      n205 = call <vilib>:"Simple Error Handler.vi"("error in (no error)"=w69) -> ()  [unwired: 4 in, 5 out]
    }
    frame True {
      w560 = "SYST:LOC\n"  # Local Command
      n206 = VISA Write(VISA resource name=w562, write buffer=w560, error in (no error)=w561) -> (VISA resource name out=w564:refnum<visa-resource-name>, error out=w563:errorcluster)  [unwired: 1 out]
      n207 = call "Error Query.vi"("error in (no error)"=w563, "VISA resource name"=w564) -> ("error out"=→"error out":errorcluster, "VISA resource name out"=→"VISA resource name out":refnum<visa-resource-name>)  [unwired: 6 in, 2 out]
      n208 = VISA Open(error in (no error)=w554, VISA resource name=w555) -> (error out=w559:errorcluster)  [unwired: 3 in, 1 out]
      n209 = VISA Write(VISA resource name=w555, write buffer="*RST" ("数据"), error in (no error)=w559) -> (error out=w558:errorcluster)  [unwired: 2 out]
      n210 = VISA Write(VISA resource name=w555, write buffer="SYST:LOC" ("address string"), error in (no error)=w558) -> (VISA resource name out=w552:refnum<visa-resource-name>, error out=w551:errorcluster)  [unwired: 1 out]
      n211 = VISA Close(VISA resource name=w552, error in (no error)=w551) -> (error out=→"error out 5":errorcluster)
    }
  }
